vi "Actor Core.vi"(8 "error in":errorcluster, 11 "Device in":refnum<class "Device.lvclass">) -> (0 "error out":errorcluster, 3 "Actor out":refnum<class "Actor.lvclass">)   [LabVIEW 2015, in "DAQ Device.lvlib" / "Device.lvclass"]
doc: "(<B>Filename</B>: Actor Framework.lvlib:Actor.lvclass:Actor Core.vi)\n\nReceives messages to the actor, reacts to them, and initiates any error handling that may shut the actor down.\n\nDescendant classes may override this VI to append parallel tasks for the actor to complete while it handles messages. Overrides use the Call Parent Method node."
uses:
  Device.lvclass
  <vilib>/ActorFramework/Actor/Actor.lvclass
  <vilib>/MSR Consulting, LLC/General Reuse/SuperActor/SuperActor.lvclass
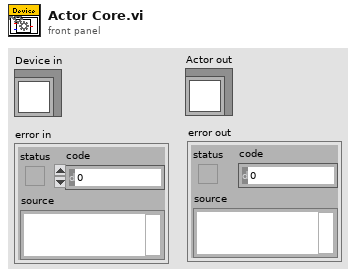
[diagram p1: front panel]
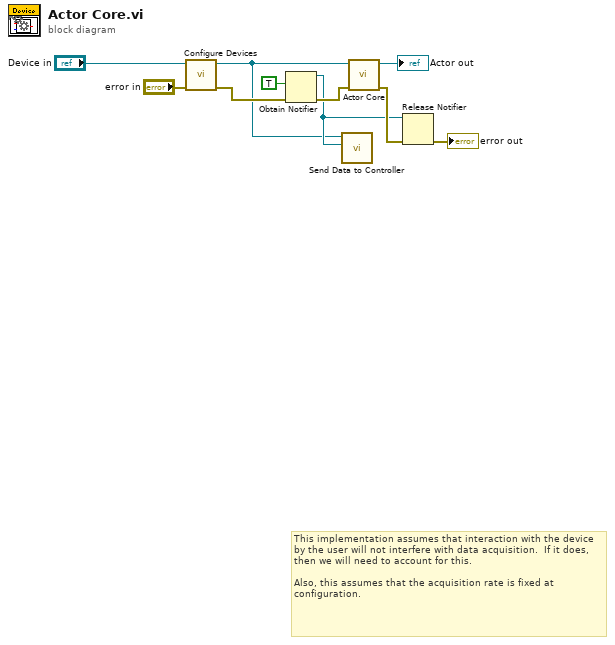
[diagram p0: block diagram]
diagram:
  # "This implementation assumes that interaction with the device by the user will not interfere with data acquisition.  If it does, then we will need to account for this.\n\nAlso, this assumes that the acquisition rate is fixed at configuration."
  n1 = call "Configure Devices.vi"("error in"="error in", "Device in"="Device in") -> ("error out"=w3:errorcluster, "Device out"=w1:refnum<class "Device.lvclass">)  [unwired: 8 in]
  n2 = Obtain Notifier(notification data type=TRUE, error in (no error)=w3) -> (notifier out=w6:refnum<notifier>, error out=w9:errorcluster)  [unwired: 2 in, 1 out]
  n3 = call "Send Data to Controller.vi"("notifier in"=w6, "Device in"=w1) -> ()  [unwired: 10 in]
  n4 = call-parent "Actor Core.vi"("error in"=w9, "Actor in"=w1) -> ("error out"=w8:errorcluster, "Actor out"=→"Actor out":refnum<class "Actor.lvclass">)  [unwired: 8 in]
  n5 = Release Notifier(notifier=w6, error in (no error)=w8) -> (error out=→"error out":errorcluster)  [unwired: 1 in, 2 out]
